vi "Write settings.vi"(8 "error in (no error)":errorcluster, 10 "settings name in":string, 11 "Cobolt in":refnum<class "Cobolt.lvclass">) -> (0 "error out":errorcluster, 2 "settings name out":string, 3 "Cobolt out":refnum<class "Cobolt.lvclass">)   [LabVIEW 2012, in "Cobolt.lvclass"]
doc: "Writes the settings cluster into the settings file. Settings file is XML-based. It's name is <component ID>.xml"
uses:
  Cobolt.lvclass
  <vilib>/Distrio/Murmex/Murmex/Murmex.lvclass
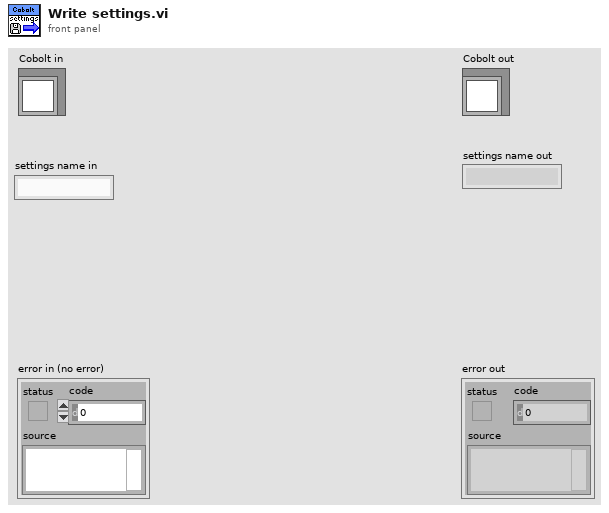
[diagram p1: front panel]
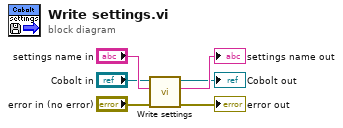
[diagram p0: block diagram]
diagram:
  n1 = call-parent "Write settings.vi"("error in (no error)"="error in (no error)", "settings name in"="settings name in", "Murmex in"="Cobolt in") -> ("error out"=→"error out":errorcluster, "settings name out"=→"settings name out":string, "Murmex out"=→"Cobolt out":refnum<class "Cobolt.lvclass">)  [unwired: 6 in]
